vi "XIPIN_AXI_Video_Direct_Memory_Access_5_04_a.vi"   [LabVIEW 2017]
doc: "The Xilinx AXI Video DMA LogiCORE provides a flexible interface for controlling and synchronizing video frame stores from external memory. Multiple VDMAs from different clock domains can be linked together to control frame store reads and writes from multiple sources. Automatic frame skips and repeats are performed to seamlessly allow frame rate conversion. Support for up to 32 external frame stores with image sizes of 4k x4k is provided. The core is programmable through a comprehensive register interface for setting and controlling frame synchronization (can be turned on/off in real-time), frame read/write delays, source synchronization switching, circular buffer enable and more using logic or a microprocessor. Frame count, delay count, and error interrupt status bits provided for processor monitoring.\n------------------------------------\n<b>Need License</b> : No\n<b>Interface</b> : AXI4 AXI4-Stream AXI4-Lite"
uses:
  <vilib>/rvi/XilinxIP/XIPIN_XNode/niFpgaXIPIN.xnode
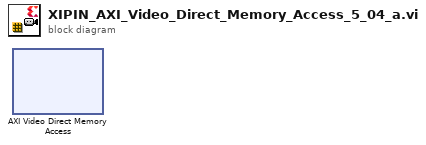
[diagram p0: block diagram]
diagram:
  n1 = xnode ("AXI Video Direct Memory Access")() -> ()
